vi "testtest.vi"(7 "Width":u32, 8 "error in (no error)":errorcluster, 9 "ValueU32 2":u32, 10 "ValueU32":u32, 11 "Refnum in":T1) -> (0 "error out":errorcluster, 3 "Codec Names":string[](array[string]))   [LabVIEW 2023]
uses:
  <vilib>/vision/Avi.llb/IMAQ AVI2 Codec Path.ctl
  <vilib>/vision/Image Controls.llb/IMAQ Image.ctl
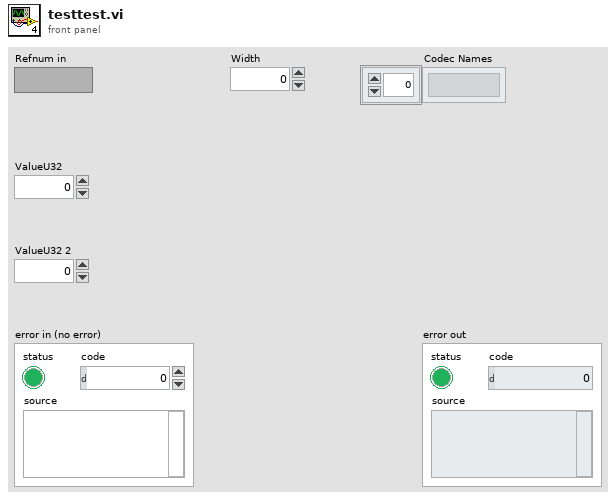
[diagram p1: front panel]
types:
  T1 = typedef "IMAQ Image.ctl" = refnum<image>
  T2 = typedef "IMAQ AVI2 Codec Path.ctl" = u32
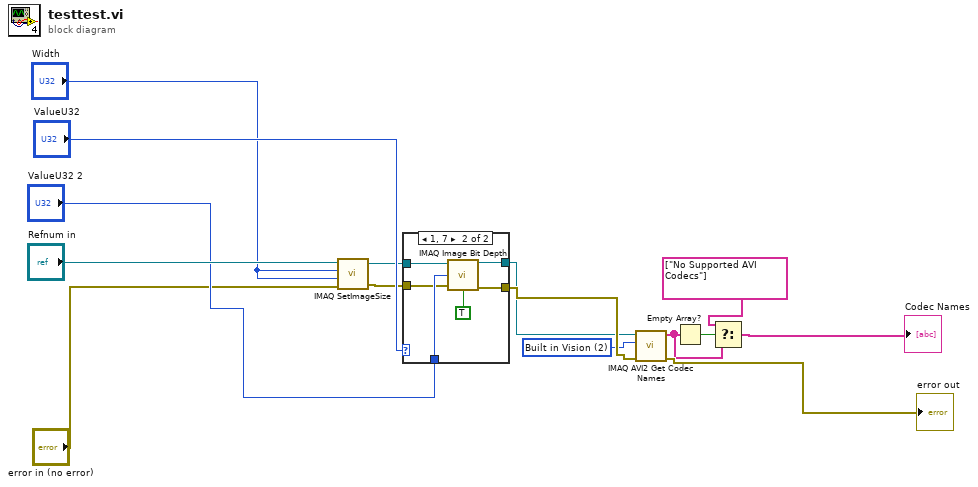
[diagram p0: block diagram]
diagram:
  w11 = T2 2 items=["Default", "System", "Built in Vision"] ("Codec Source")
  n1 = call "IMAQ SetImageSize"("error in (no error)"="error in (no error)", "Y Resolution"="Width", "X Resolution"="Width", "Image"="Refnum in") -> ("error out"=w4:errorcluster, "Image Out"=w3:T1)  [unwired: 1 in]
  n2 = case shown="1, 7" "ValueU32" {
    tunnel: [w16 w23] -> w12
    tunnel: "ValueU32 2" -> [_ w22]
    tunnel: w4 -> [w16 w21]
    tunnel: w3 -> [w17 w19]
    tunnel: [w17 w18] -> w10
    frame 0, Default {
    }
    frame 1, 7 {
      n3 = call "IMAQ Image Bit Depth"("Image"=w19, "Bit Depth (0)"=w22, "error in (no error)"=w21, "Get/Set Bit Depth? (Set)"=TRUE) -> ("Image Out"=w18:T1, "error out"=w23:errorcluster)  [unwired: 9 in, 1 out]
    }
  }
  n4 = call "IMAQ AVI2 Get Codec Names"("error in (no error)"=w12, "Codec Source"=w11, "Image"=w10) -> ("error out"=→"error out":errorcluster, "Codec Names"=w7:string[])  [unwired: 7 in]
  n5 = Empty Array?(array=w7) -> (empty?=w8:bool)
  n6 = Select(t=string[] ["No Supported AVI Codecs"], s=w8, f=w7) -> (s? t:f=→"Codec Names":string[])
